vi "Read Caller Enqueuer (Wrap).vi"(11 "CO2 Actor in":refnum<class "CO2 Actor.lvclass">) -> (2 "Actor Framework:Message Enqueuer":refnum<class "Message Enqueuer.lvclass">, 3 "CO2 Actor out":refnum<class "CO2 Actor.lvclass">)   [LabVIEW 2015, in "cRIO-Carbondioxide.lvlib" / "CO2-Actor.lvlib" / "CO2 Actor.lvclass"]
uses:
  CO2 Actor.lvclass
  <vilib>/ActorFramework/Message Enqueuer/Message Enqueuer.lvclass
  <vilib>/ActorFramework/Actor/Actor.lvclass
  <vilib>/ActorFramework/Actor/Actor.lvclass/Actor.ctl
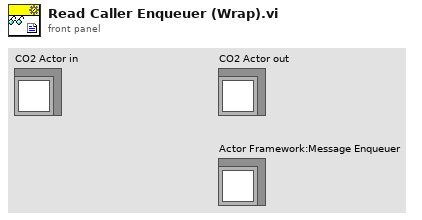
[diagram p1: front panel]
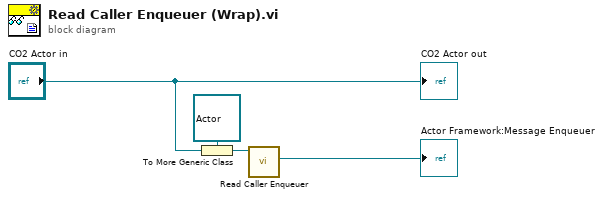
[diagram p0: block diagram]
diagram:
  n1 = To More Generic Class(target class=refnum<class "Actor.lvclass"> refnum ("Actor"), reference="CO2 Actor in") -> (generic class reference=w2:refnum<class "Actor.lvclass">)
  n2 = call <vilib>:"Read Caller Enqueuer.vi"("Actor"=w2) -> ("Caller Enqueuer"=→"Actor Framework:Message Enqueuer":refnum<class "Message Enqueuer.lvclass">)  [unwired: 10 in]
  "CO2 Actor out" <- "CO2 Actor in"
